vi "tm_frameaveraging.vi"(8 "error in (no error)":errorcluster, 10 "Frames":i32(ring)=2 items=["1 Frame"=1, "2 Frames"=2, "4 Frames"=4, "8 Frames"=8, "16 Frames"=16], 11 "Handle in":u32) -> (0 "error out":errorcluster, 3 "Handle out":u32)   [LabVIEW 2012]
uses:
  tmcamcon.dll
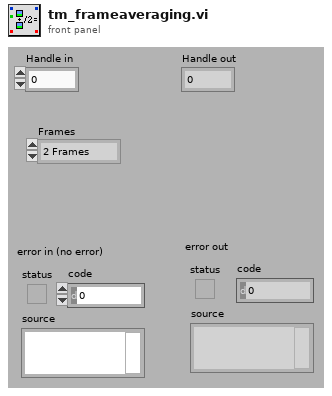
[diagram p1: front panel]
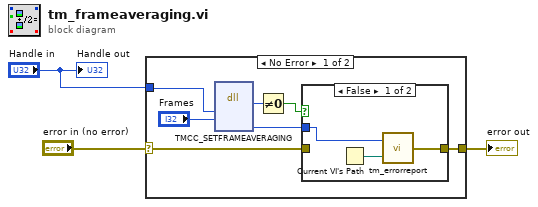
[diagram p0: block diagram]
diagram:
  n1 = case shown="No Error" "error in (no error)" {
    selector: "error in (no error)" -> [w7 w15]
    tunnel: [w4 w15] -> w2
    tunnel: "Handle in" -> [w8 _]
    frame No Error {
      n2 = dll-call lib="tmcamcon.dll" fn="TMCC_SETFRAMEAVERAGING"("HDCAM"=w8, "frames"="Frames") -> ("return type"=w10:u32, "Erval"=w6:i32)  [unwired: 6 in, 2 out]
      n3 = Not Equal To 0?(x=w10) -> (x != 0?=w5:bool)
      n4 = case shown="False" w5 {
        tunnel: w7 -> [_ w14]
        tunnel: [w12 w14] -> w4
        tunnel: w6 -> [w11 _]
        frame False {
          n5 = Current VI's Path() -> (path=w13:path)
          n6 = call "tm_errorreport.vi"("Source"=w13, "Error"=w11) -> ("error out"=w12:errorcluster)
        }
        frame True {
        }
      }
    }
    frame Error {
    }
  }
  "error out" <- w2
  "Handle out" <- "Handle in"
